vi "428_MEAS (SubVI).vi"(2 "Measurement Command":T1(ring), 3 "Response Format":enum16{"Scalar", "Array"}(ring), 4 "Measurement Type":enum16{"Measure", "Read", "Fetch"}(ring)) -> (0 "String":string, 1 "Input string 2":string)   [LabVIEW 2016]
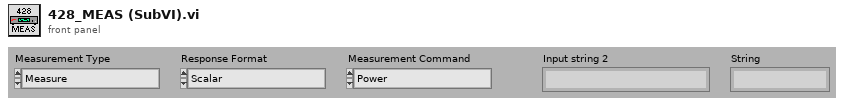
[diagram p1: front panel]
types:
  T1 = enum16{"Power", "Environment", "Wavelength", "Wave Number", "Frequency"}
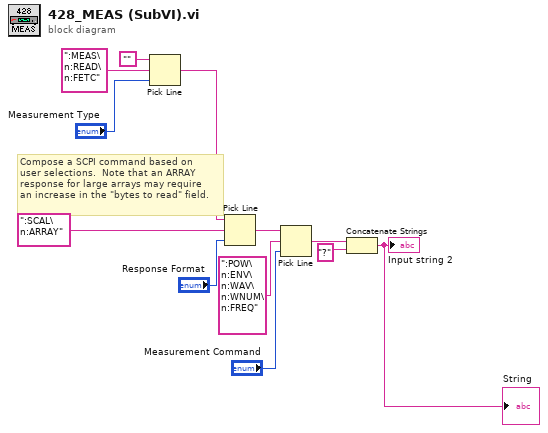
[diagram p0: block diagram]
diagram:
  # "Compose a SCPI command based on\nuser selections.  Note that an ARRAY\nresponse for large arrays may require\nan increase in the \"bytes to read\" field."
  n1 = Pick Line(string ("")="", multi-line string=":MEAS\n:READ\n:FETC", line index="Measurement Type") -> (output string=w11:string)
  n2 = Pick Line(string ("")=w11, multi-line string=":SCAL\n:ARRAY", line index="Response Format") -> (output string=w5:string)
  n3 = Pick Line(string ("")=w5, multi-line string=":POW\n:ENV\n:WAV\n:WNUM\n:FREQ", line index="Measurement Command") -> (output string=w3:string)
  n4 = Concatenate Strings(w3, "?") -> (→"Input string 2" →"String":string)
